vi "test5.vi"(11 "k":i32) -> (2 "output bit stream":i8[](array[numeric]), 3 "Array":dbl[](array[numeric]))   [LabVIEW 2018]
uses:
  <vilib>/addons/Modulation/niDMT.lvlib
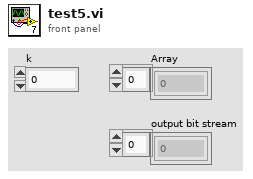
[diagram p1: front panel]
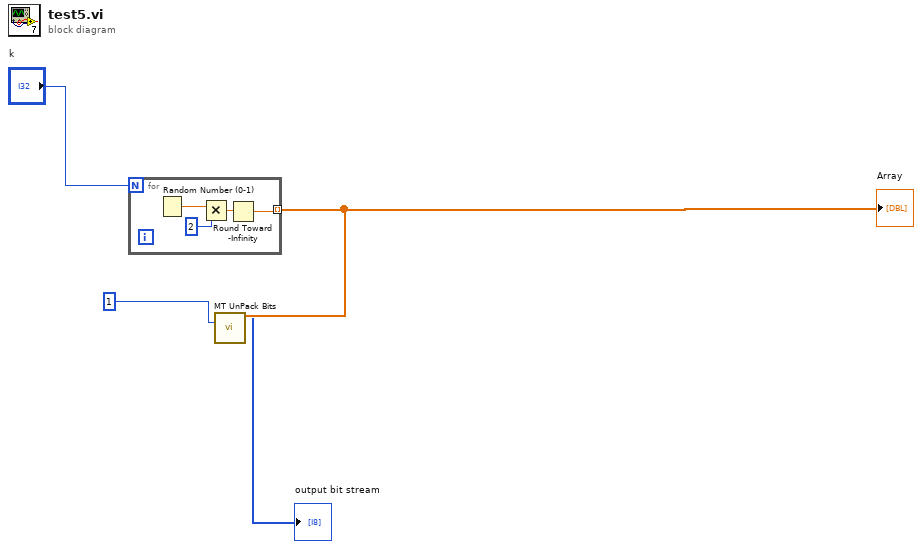
[diagram p0: block diagram]
diagram:
  n1 = for {
    N: "k" -> [_]
    tunnel: [w5] -> w4 mode=indexing
    n2 = Random Number (0-1)() -> (number: 0 to 1=w8:dbl)
    n3 = Multiply(x=w8, y=2) -> (x*y=w6:dbl)
    n4 = Round Toward -Infinity(1:w6) -> (0:w5:dbl)
  }
  "Array" <- w4
  n5 = call <vilib>:"MT UnPack Bits.vi"("input integers"=w4, "bits per integer"=1) -> ("output bit stream"=→"output bit stream":i8[])  [unwired: 12 in, 1 out]
